vi "uMsg Get Payload.vi"(8 "error in (no error)":errorcluster, 11 "uMsg in":refnum<class "uMsg.lvclass">) -> (0 "error out":errorcluster, 2 "uData":refnum<class "uData.lvclass">, 3 "uMsg out":refnum<class "uMsg.lvclass">)   [LabVIEW 2023, in "uFramework.lvlib" / "uMsg.lvclass"]
uses:
  uMsg.lvclass
  Bin/uData.lvlibp/uData.lvclass
  uMsg.lvclass/uMsg.ctl
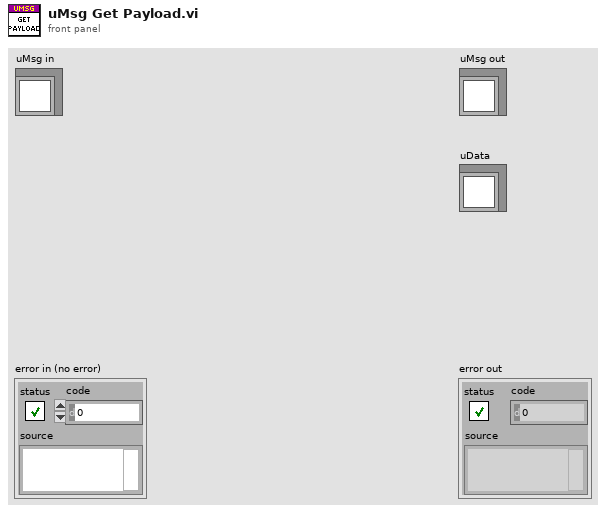
[diagram p1: front panel]
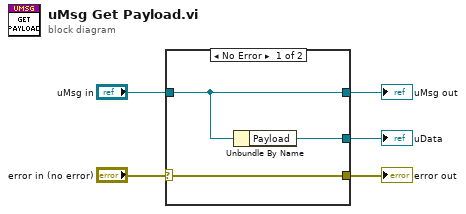
[diagram p0: block diagram]
diagram:
  n1 = case shown="No Error" "error in (no error)" {
    selector: "error in (no error)" -> [w6 w9]
    tunnel: [w8 _] -> w5
    tunnel: "uMsg in" -> [w7 w10]
    tunnel: [w7 w10] -> w3
    tunnel: [w6 w9] -> w1
    frame No Error {
      n2 = Unbundle By Name(w7) -> ("Payload"=w8:refnum<class "uData.lvclass">)
    }
    frame Error {
    }
  }
  "error out" <- w1
  "uMsg out" <- w3
  "uData" <- w5
